vi "Route Parameter String.vi"(8 "error in (no error)":errorcluster, 9 "Output Index":i32, 10 "Input Index":i32, 11 "Voicemeeter Type":T1) -> (0 "error out":errorcluster, 2 "Route Parameter String":string)   [LabVIEW 2020, in "VoiceMeeterRemote.lvlib" / "VoiceMeeterRemote.lvclass"]
uses:
  VoiceMeeterRemote.lvclass
  Voicemeeter Type.ctl
  VoiceMeeterRemote.lvlib
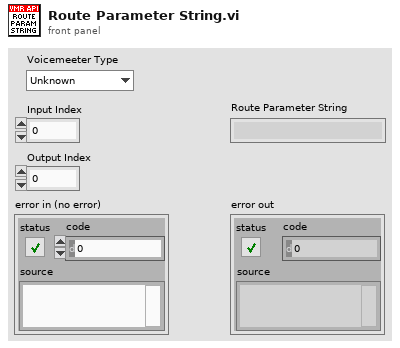
[diagram p1: front panel]
types:
  T1 = typedef "VoiceMeeterRemote.lvlib/Voicemeeter Type.ctl" = enum16{"Unknown", "Voicemeeter", "Banana", "Potato", "Potato x64"}
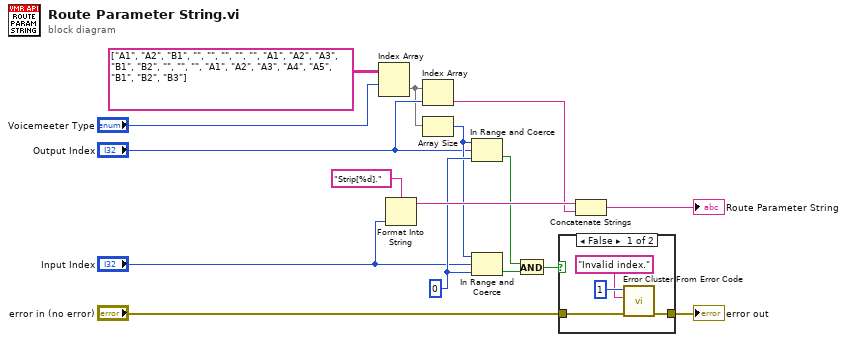
[diagram p0: block diagram]
diagram:
  w12 = 0 ("lower limit")
  n1 = Index Array(array=string[][] [["A1", "A2", "B1", "", "", "", "", ""], ["A1", "A2", "A3", "B1", "B2", "", "", ""], ["A1", "A2", "A3", "A4", "A5", "B1", "B2", "B3"]], index (row)="Voicemeeter Type") -> (element=w5:string[])  [unwired: 1 in]
  n2 = Format Into String(format string="Strip[%d].", "Input Index") -> (resulting string=w15:string)  [unwired: 2 in, 1 out]
  n3 = Index Array(array=w5, index="Output Index") -> (element=w10:string)
  n4 = Array Size(array=w5) -> (size(s)=w11:i32)
  n5 = In Range and Coerce(upper limit=w11, x="Output Index", lower limit=w12) -> (In Range?=w13:bool)  [unwired: 1 out]
  n6 = In Range and Coerce(upper limit=w11, x="Input Index", lower limit=w12) -> (In Range?=w9:bool)  [unwired: 1 out]
  n7 = And(x=w13, y=w9) -> (x .and. y?=w2:bool)
  n8 = case shown="False" w2 {
    tunnel: "error in (no error)" -> [w20 w21]
    tunnel: [w19 w21] -> w1
    frame False {
      n9 = call <vilib>:"Error Cluster From Error Code.vi"("error in (no error)"=w20, "error message (\"\")"="Invalid index.", "error code (0)"=1) -> ("error out"=w19:errorcluster)  [unwired: 6 in]
    }
    frame True {
    }
  }
  "error out" <- w1
  n10 = Concatenate Strings(w15, w10) -> (→"Route Parameter String":string)
